vi "配置属性操作.vi"(6 "error in (no error)":errorcluster caption="错误输入（无错误）", 9 "引用":refnum<vi>) -> (0 "error out":errorcluster caption="错误输出", 3 "配置提取集合":T1)   [LabVIEW 2017]
uses:
  <vilib>/Utility/file.llb/Read Delimited Spreadsheet (string).vi
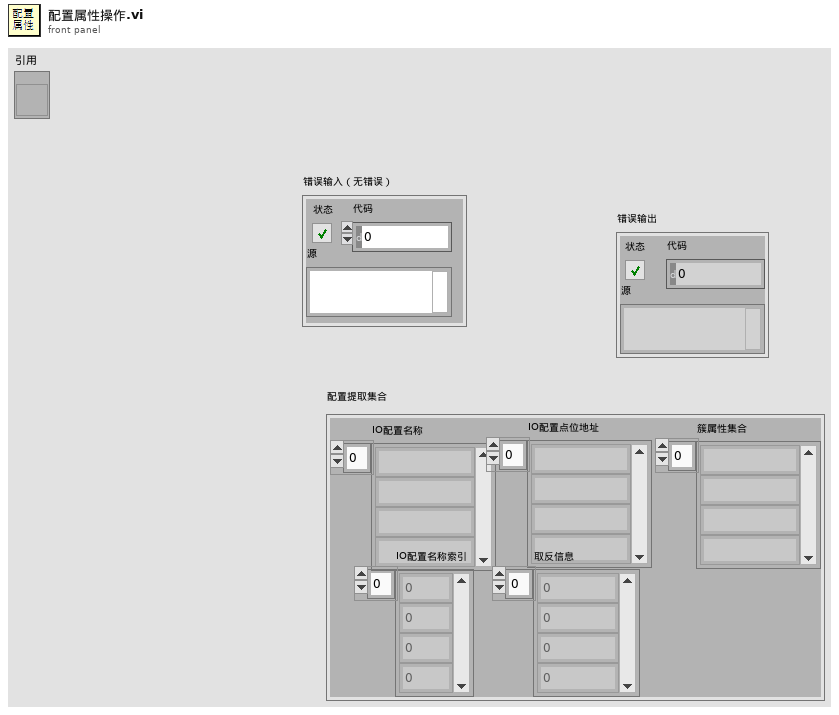
[diagram p1: front panel]
types:
  T1 = typedef "输入&输出配置提取集合.ctl" = cluster{"IO配置名称":string[], "IO配置点位地址":string[], "IO配置名称索引":i32[], "取反信息":i32[], "簇属性集合":string[]}
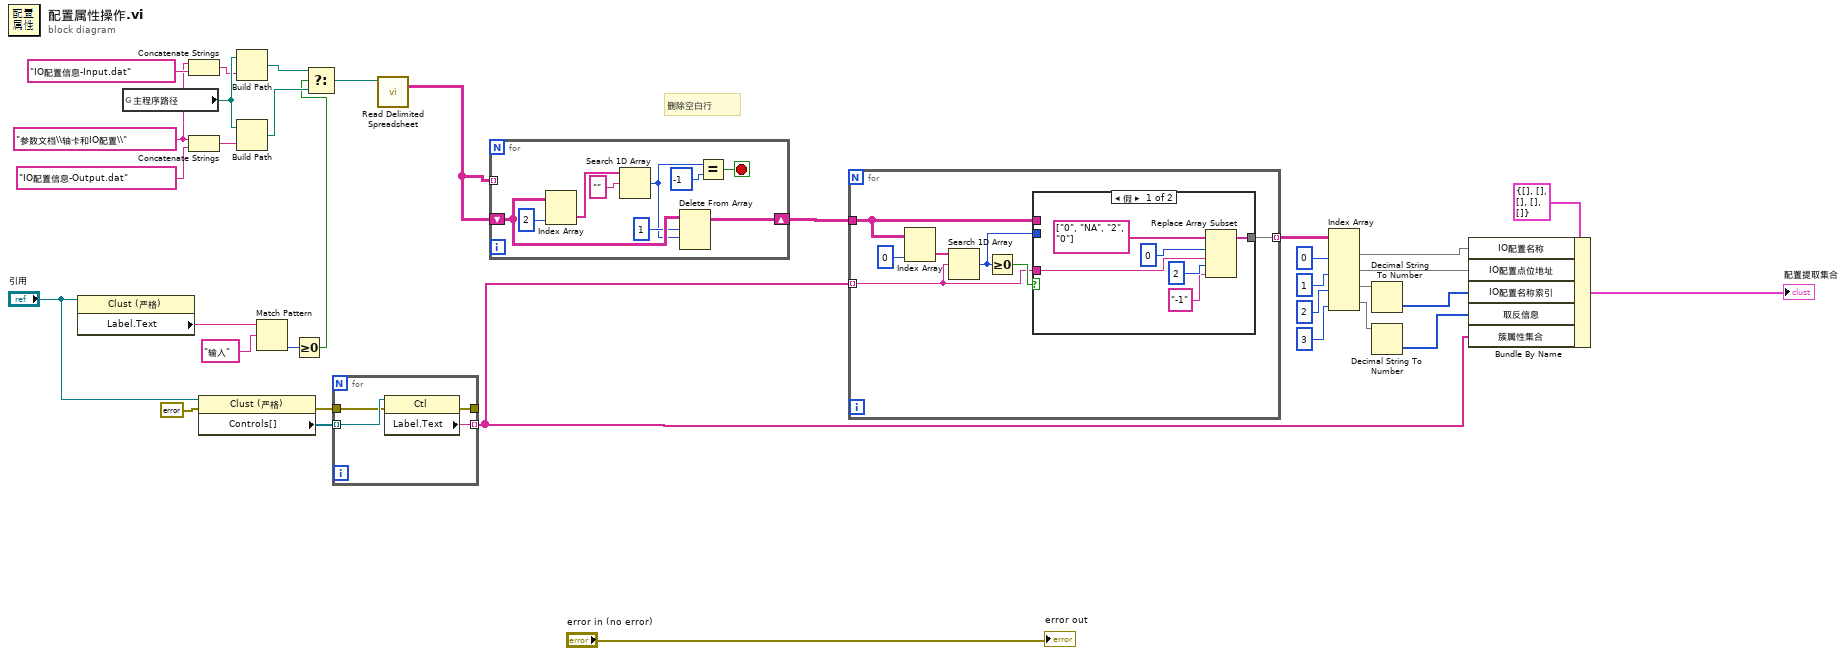
[diagram p0: block diagram]
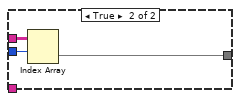
[diagram p2: hidden frame]
diagram:
  w9 = "参数文档\\轴卡和IO配置\\" ("名称或相对路径")
  # "删除空白行"
  n1 = property on="属性节点" class="Clust (严格)"(reference="引用") -> ("Label.Text"=w14:string)  [unwired: 1 in, 2 out]
  n2 = global read "全局 1.vi" "主程序路径"() -> (w31:path)
  n3 = Concatenate Strings(w9, "IO配置信息-Input.dat" ("名称或相对路径")) -> (w10:string)
  n4 = Concatenate Strings(w9, "IO配置信息-Output.dat" ("名称或相对路径")) -> (w7:string)
  n5 = property on="属性节点" class="Clust (严格)"(reference="引用", error in=errorcluster {"status"=FALSE, "code"=0, "source"=""} ("错误输入（无错误）")) -> (error out=w32:errorcluster, "Controls[]"=w33:refnum<vi>[])  [unwired: 1 out]
  n6 = Build Path(base path=w31, name or relative path=w10) -> (appended path=w5:path)
  n7 = Build Path(base path=w31, name or relative path=w7) -> (appended path=w4:path)
  n8 = Match Pattern(string=w14, regular expression="输入" ("正则表达式")) -> (offset past match=w12:i32)  [unwired: 1 in, 3 out]
  n9 = Greater Or Equal To 0?(x=w12) -> (x >= 0?=w3:bool)
  n10 = Select(t=w5, s=w3, f=w4) -> (s? t:f=w6:path)
  n11 = for {
    tunnel: w33 -> [w38] mode=indexing
    tunnel: w32 -> [w37]
    tunnel: [w36] -> _
    tunnel: [w35] -> w16 mode=indexing
    n12 = property class="Ctl"(reference=w38, error in=w37) -> (error out=w36:errorcluster, "Label.Text"=w35:string)  [unwired: 1 out]
  }
  n13 = call-poly <vilib>:"Read Delimited Spreadsheet.vi"("file path (dialog if empty)"=w6) -> ("all rows"=w2:string[][])  [unwired: 9 in, 5 out]
  n14 = for {
    shift-right: [w41] -> w30
    shift-left: w2 -> [w42]
    tunnel: w2 -> [_] mode=indexing
    stop <- w43 stop-if-true
    n15 = Index Array(array=w42, index (col)=2 ("禁用的索引 (列)")) -> (element=w46:string[])  [unwired: 1 in]
    n16 = Search 1D Array(1D array=w46, element="" ("元素")) -> (index of element=w39:i32)  [unwired: 1 in]
    n17 = Delete From Array(array=w42, length=1 ("长度"), index (row)=w39) -> (array with subset deleted=w41:string[][])  [unwired: 1 in, 1 out]
    n18 = Equal?(x=w39, y=-1) -> (x = y?=w43:bool)
  }
  n19 = for {
    tunnel: w16 -> [w52] mode=indexing
    tunnel: w30 -> [w50]
    tunnel: [w51] -> w29 mode=indexing
    n20 = Index Array(array=w50, index (col)=0 ("禁用的索引 (列)")) -> (element=w48:string[])  [unwired: 1 in]
    n21 = Search 1D Array(1D array=w48, element=w52) -> (index of element=w54:i32)  [unwired: 1 in]
    n22 = Greater Or Equal To 0?(x=w54) -> (x >= 0?=w53:bool)
    n23 = case shown="假" w53 {
      tunnel: w50 -> [_ w63]
      tunnel: w54 -> [_ w62]
      tunnel: [w59 w61] -> w51
      tunnel: w52 -> [w57 _]
      frame False {
        n24 = Replace Array Subset(array=string[] ["0", "NA", "2", "0"] ("all rows"), new element #1=w57, index #1=0 ("索引"), new element #2="-1" ("新元素/子数组"), index #2=2 ("索引")) -> (w59:string[])
      }
      frame True {
        n25 = Index Array(array=w63, index (row)=w62) -> (element=w61:string[])  [unwired: 1 in]
      }
    }
  }
  n26 = Index Array(array=w29, index (col) #1=0 ("禁用的索引 (列)"), index (col) #2=1 ("索引 (列)"), index (col) #3=2 ("索引 (列)"), index (col) #4=3 ("索引 (列)")) -> (element #1=w22:string[], element #2=w21:string[], element #3=w20:string[], element #4=w18:string[])  [unwired: 4 in]
  n27 = Decimal String To Number(string=w20) -> (number=w19:i32[])  [unwired: 2 in, 1 out]
  n28 = Decimal String To Number(string=w18) -> (number=w17:i32[])  [unwired: 2 in, 1 out]
  n29 = Bundle By Name(cluster=T1 {"IO配置名称"=[], "IO配置点位地址"=[], "IO配置名称索引"=[], "取反信息"=[], "簇属性集合"=[]} ("输出配置提取集合"), "IO配置名称"=w22, "IO配置点位地址"=w21, "IO配置名称索引"=w19, "取反信息"=w17, "簇属性集合"=w16) -> (→"配置提取集合":T1)
  "error out" <- "error in (no error)"
